vi "SA40144C.20210105.vi"() -> ()   [LabVIEW 2020]
uses:
  <vilib>/Analysis/baseanly.llb/Mean (DBL).vi
  <userlib>/LevyLab/LV to ITX/Data/Data.lvclass
  <userlib>/LevyLab/XY Utilities/xy_utilities.lvlib
  <vilib>/Analysis/NI_AALBase.lvlib
panel:
  in  "Array":path[](array[path])=[path "G:/My Drive/ansom/Data/PPMS 2/SA40144C.20210105/01 - Vacuum Thermal Decay/SA40144C.20210105.275K.dat", path "G:/My Drive/ansom/Data/PPMS 2/SA40144C.20210105/01 - Vacuum Thermal Decay/SA40144C.20210105.280K.dat", path "G:/My Drive/ansom/Data/PPMS 2/SA40144C.20210105/01 - Vacuum Thermal Decay/SA40144C.20210105.285K.dat", path "G:/My Drive/ansom/Data/PPMS 2/SA40144C.20210105/01 - Vacuum Thermal Decay/SA40144C.20210105.295K.dat", path "G:/My Drive/ansom/Data/PPMS 2/SA40144C.20210105/01 - Vacuum Thermal Decay/SA40144C.20210105.310K.dat", path "G:/My Drive/ansom/Data/PPMS 2/SA40144C.20210105/01 - Vacuum Thermal Decay/SA40144C.20210105.315K.dat", path "G:/My Drive/ansom/Data/PPMS 2/SA40144C.20210105/01 - Vacuum Thermal Decay/SA40144C.20210105.320K.dat", path "G:/My Drive/ansom/Data/PPMS 2/SA40144C.20210105/01 - Vacuum Thermal Decay/SA40144C.20210105.325K.dat", path "G:/My Drive/ansom/Data/PPMS 2/SA40144C.20210105/01 - Vacuum Thermal Decay/SA40144C.20210105.330K.dat", path "G:/My Drive/ansom/Data/PPMS 2/SA40144C.20210105/01 - Vacuum Thermal Decay/SA40144C.20210105.335K.dat", path "G:/My Drive/ansom/Data/PPMS 2/SA40144C.20210105/01 - Vacuum Thermal Decay/SA40144C.20210105.340K.dat", path "G:/My Drive/ansom/Data/PPMS 2/SA40144C.20210105/01 - Vacuum Thermal Decay/SA40144C.20210105.345K.dat", path "G:/My Drive/ansom/Data/PPMS 2/SA40144C.20210105/01 - Vacuum Thermal Decay/SA40144C.20210105.350K.dat"]
  in  "Temps to keep (Lifespan)":i32=26
  out "Lifespan vs Temp (hrs)":cluster{i32[], dbl[]}[](graph)
  out "E_a":dbl[](array[numeric])
  out "Arrhenius":T1(graph)
  in  "Temps to keep (Arrhenius fit)":i32=26
  out "G2T vs t":T1(graph)
  out "G4T vs t":T1(graph)
  out "G2T vs t 2D":T1(graph)
  out "G4T vs t  2D":T1(graph)
  in  "Source Voltage":dbl=0.01
  in  "Init Temp":i32=275
  in  "Temp Step":i32=5
  in  "Final Temp":i32=400
  in  "Trimming":i32=400
  in  "Update":bool
  in  "OK":bool
  out "error out":errorcluster
  in  "error in (no error)":errorcluster
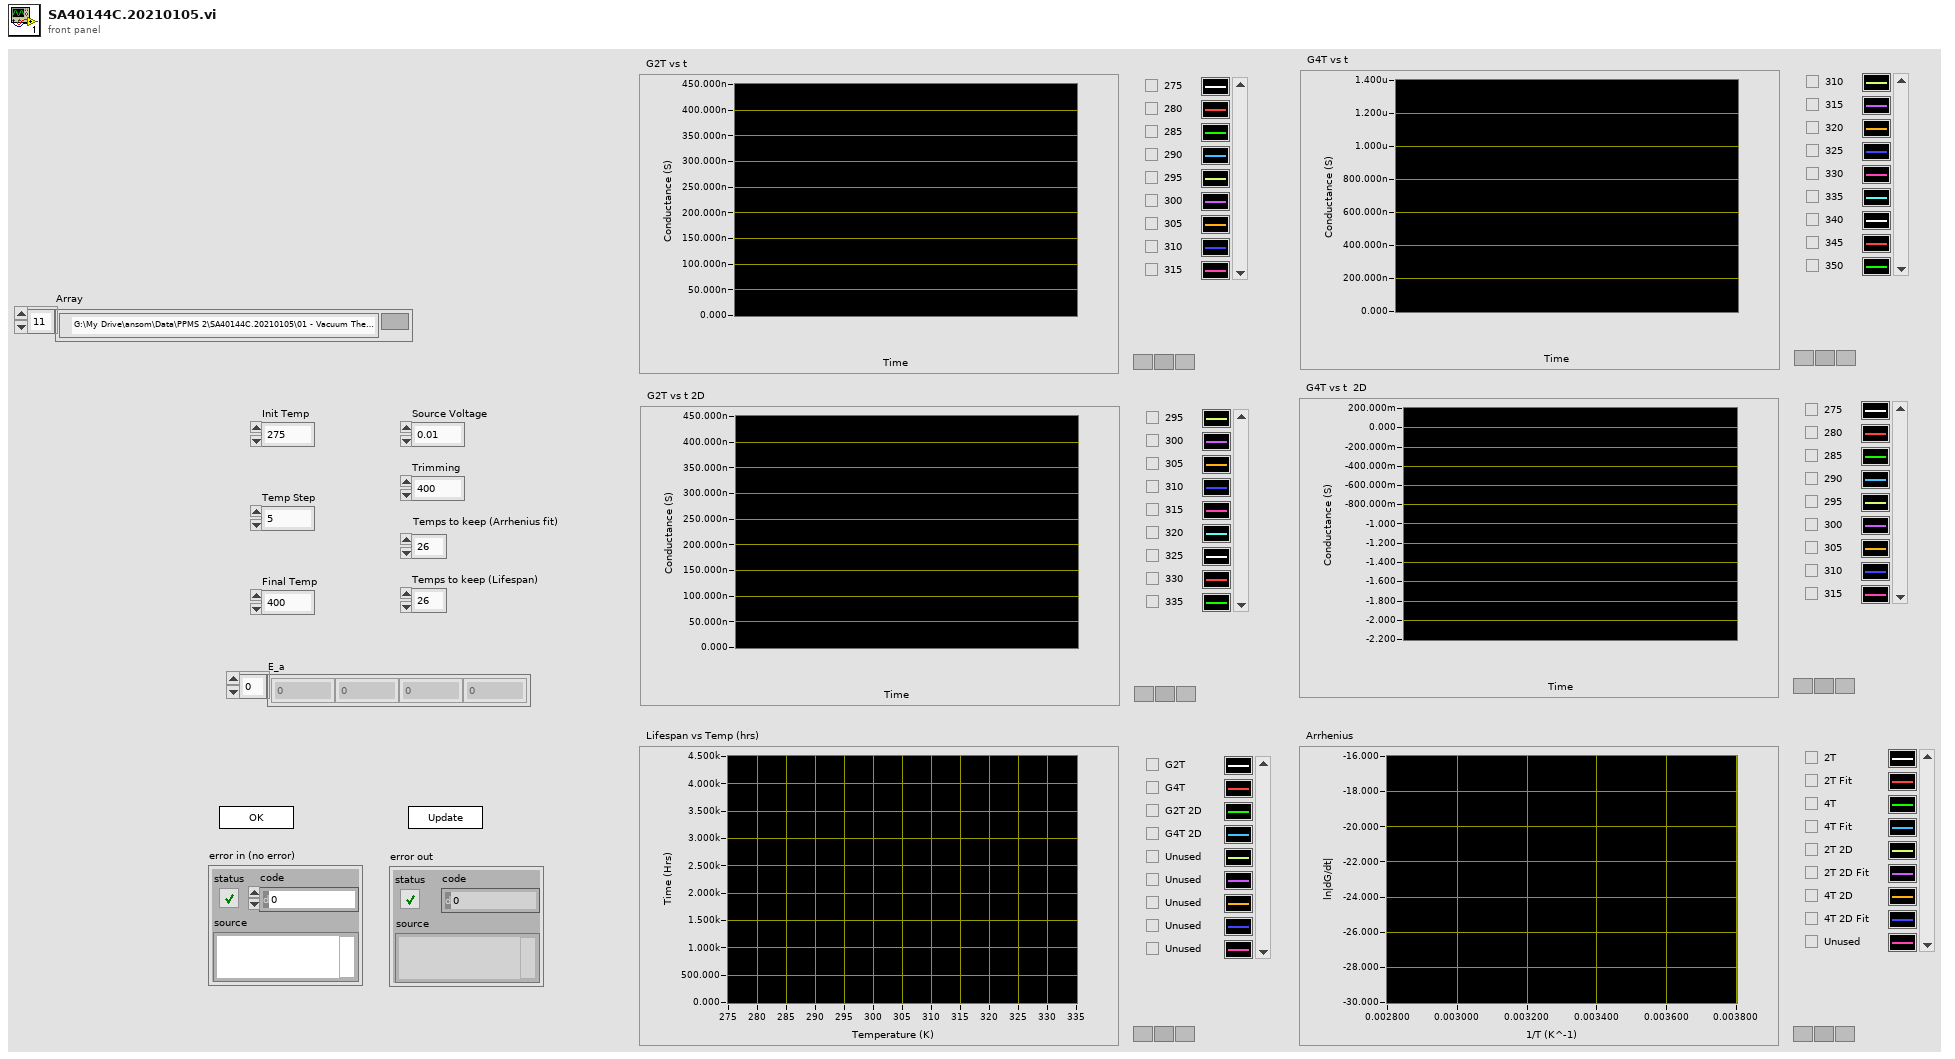
[diagram p1: front panel]
types:
  T1 = cluster{"Data":dbl[], "Best Exponential Fit":dbl[]}[]
  T2 = enum32{"Invalid", "Standard", "Closed", "Hidden", "Minimized", "Maximized"}
  T3 = enum32{"invalid app kind", "Development System", "Run Time System", "Student Edition", "Embedded LabVIEW", "Evaluation", "Custom"}
  T4 = cluster{"Core":cluster{"Current VI Reference":refnum<vi>, "Close Panel on Exit?":bool}, "G2T 1D":cluster{dbl[], dbl[]}[], "G4T 1D":cluster{dbl[], dbl[]}[], "G2T 2D":cluster{dbl[], dbl[]}[], "G4T 2D":cluster{dbl[], dbl[]}[], "Source Voltage":dbl, "Final Temp":i32, "Init Temp":i32, "Temp Step":i32, "Trimming":i32, "Array":path[], "Temp Array":dbl[]}
  T5 = cluster{"Current VI Reference":refnum<vi>, "Close Panel on Exit?":bool}
  T6 = typedef "Data.lvclass/Dictionary--cluster.ctl" = cluster{"key":string, "value":variant}
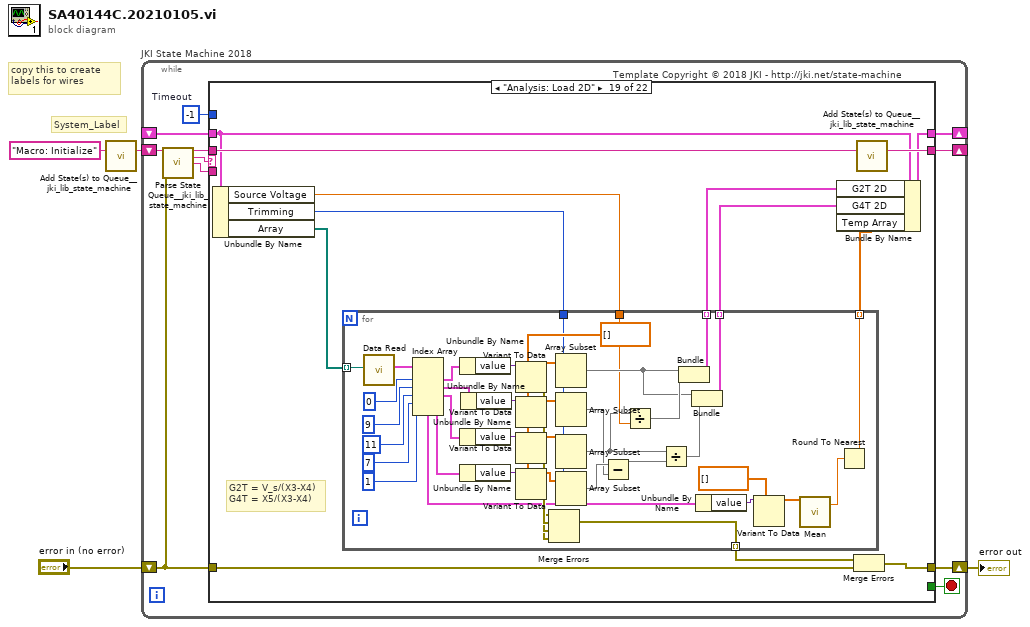
[diagram p0: block diagram]
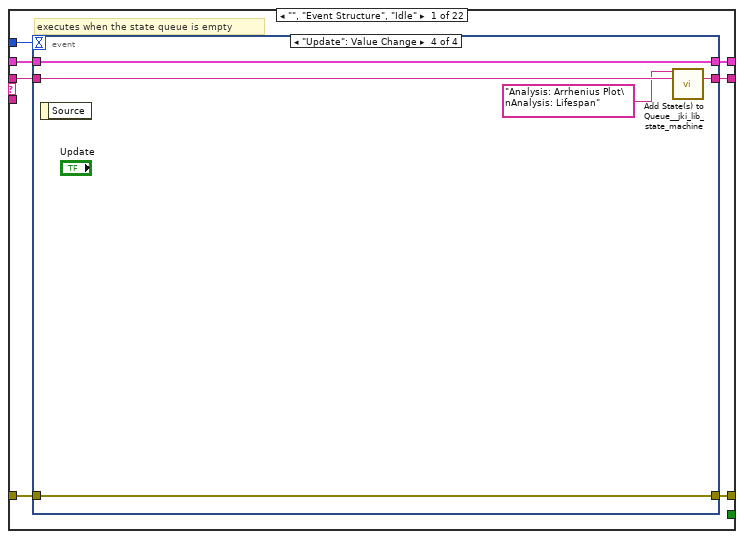
[diagram p2: hidden frame]
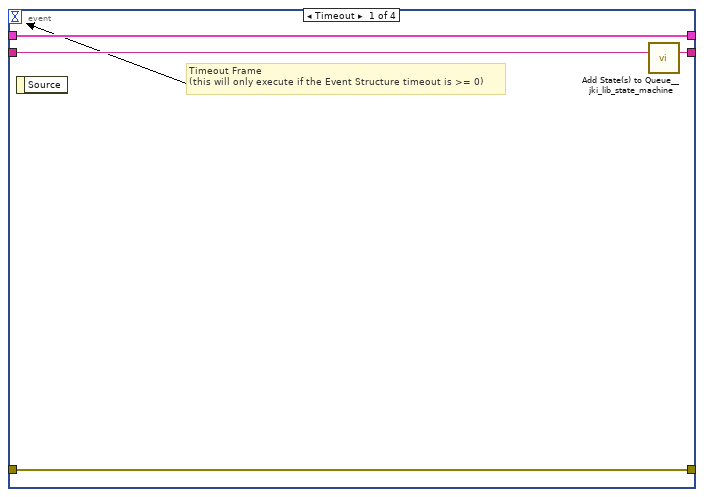
[diagram p3: hidden frame]
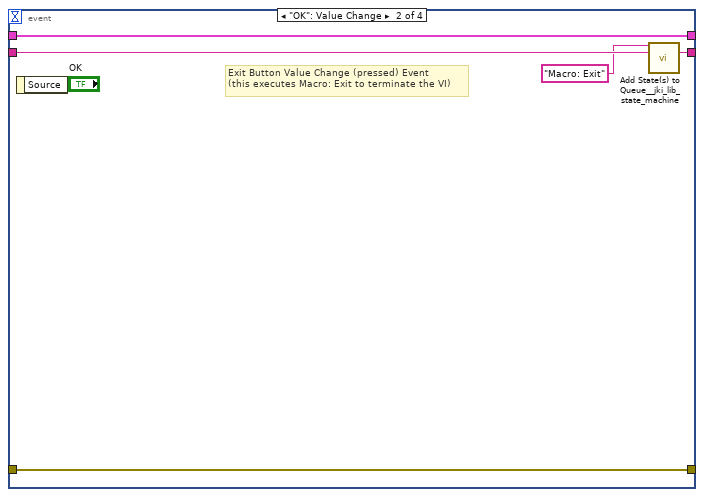
[diagram p4: hidden frame]
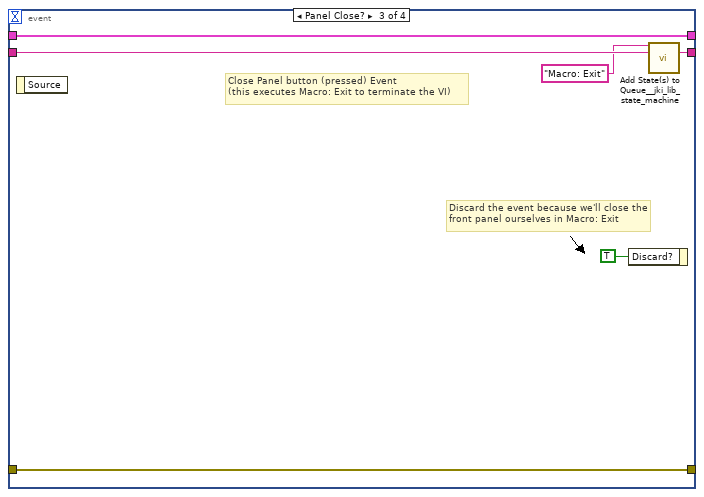
[diagram p5: hidden frame]
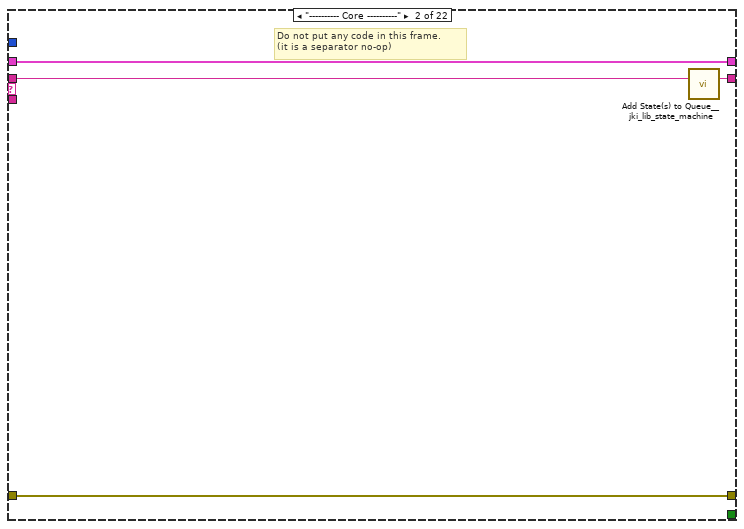
[diagram p6: hidden frame]
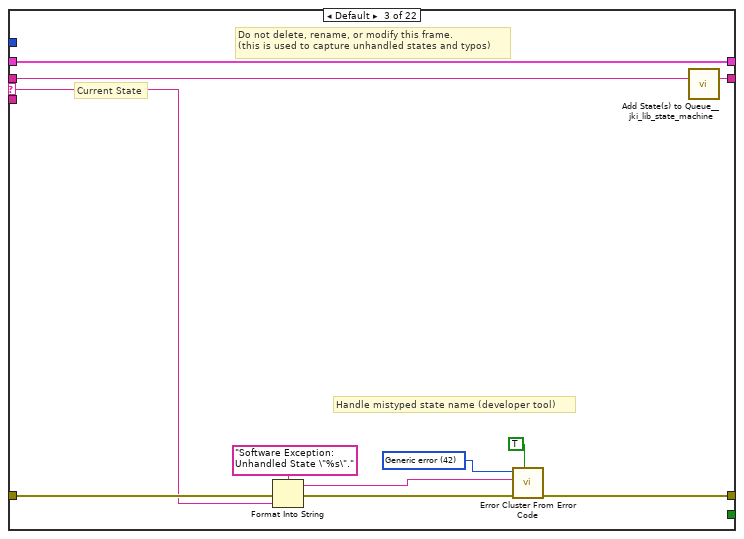
[diagram p7: hidden frame]
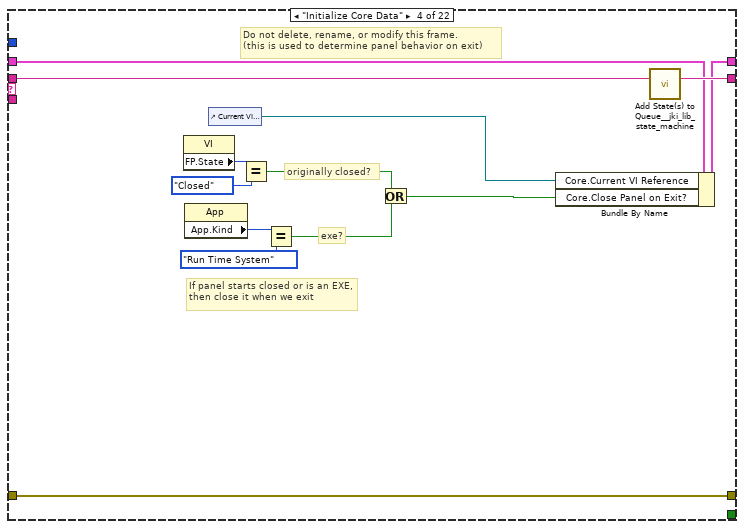
[diagram p8: hidden frame]
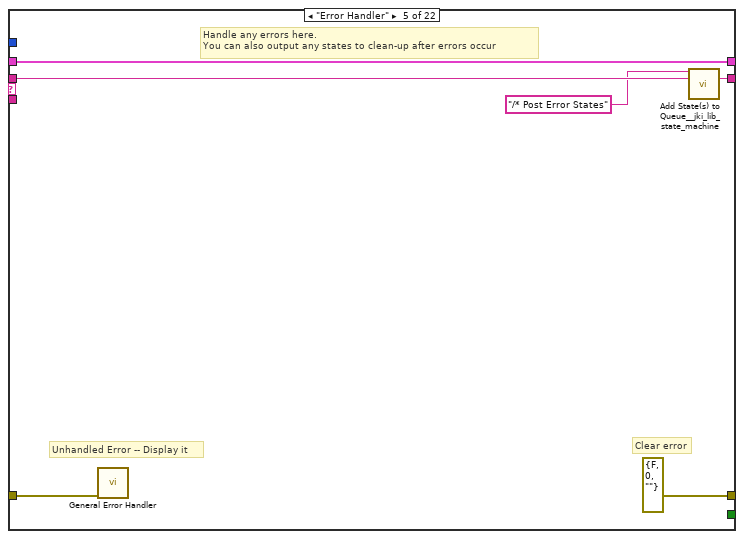
[diagram p9: hidden frame]
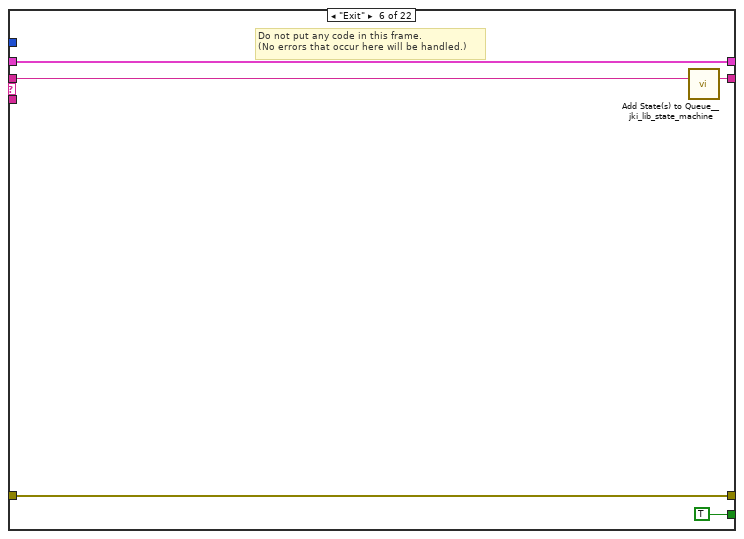
[diagram p10: hidden frame]
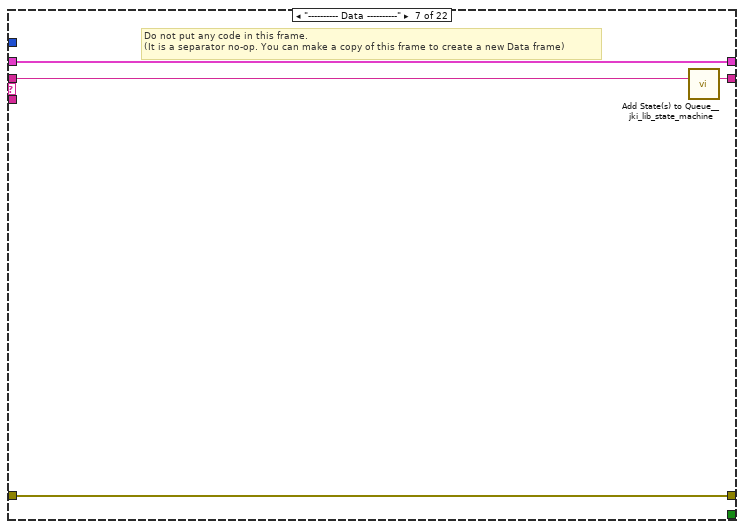
[diagram p11: hidden frame]
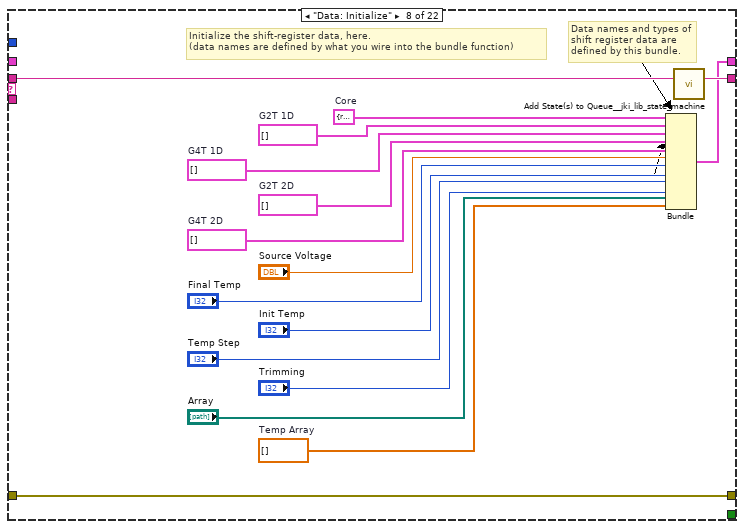
[diagram p12: hidden frame]
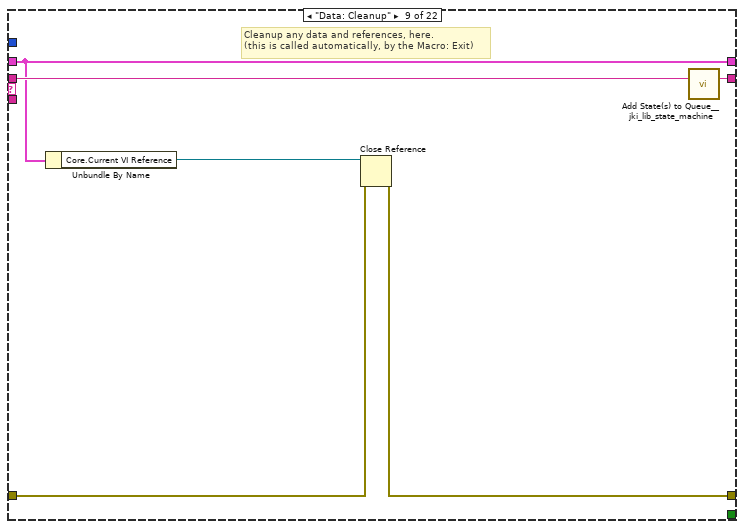
[diagram p13: hidden frame]
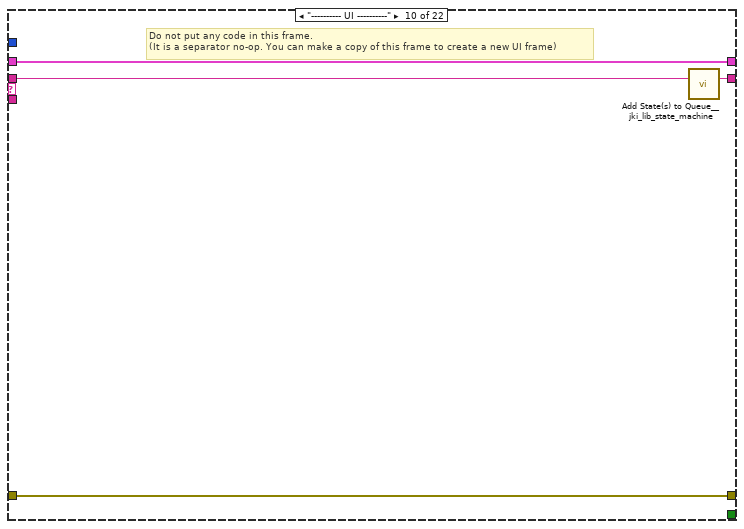
[diagram p14: hidden frame]
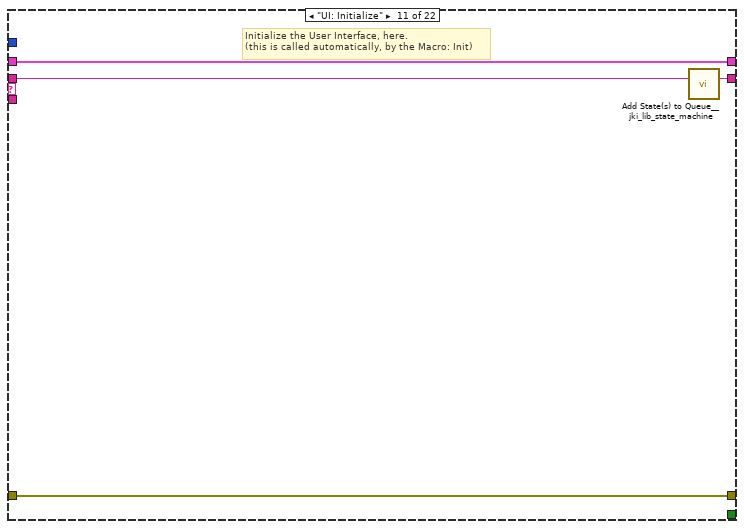
[diagram p15: hidden frame]
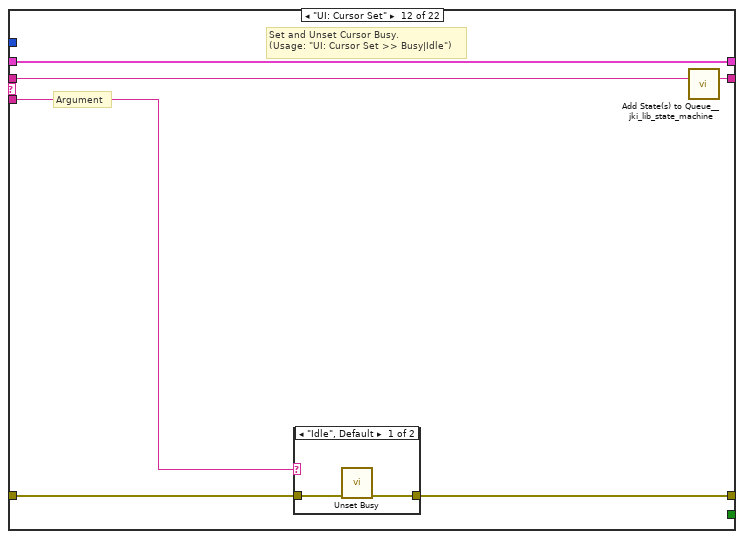
[diagram p16: hidden frame]
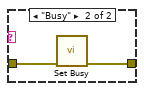
[diagram p17: hidden frame]
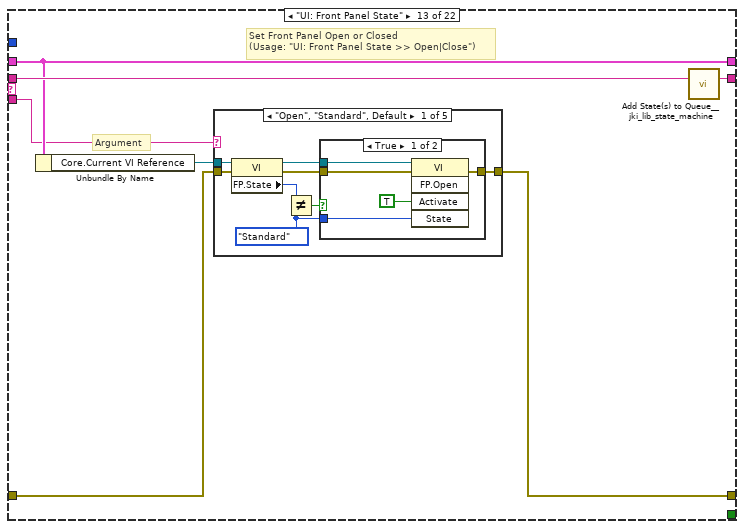
[diagram p18: hidden frame]
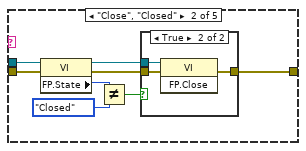
[diagram p20: hidden frame]
diagram:
  # "copy this to create labels for wires"
  # "System_Label"
  n1 = call <vilib>:"Add State(s) to Queue__jki_lib_state_machine.vi"("State(s) in (\"\")"="Macro: Initialize") -> ("States Out"=w4:string)  [unwired: 14 in]
  n2 = while "JKI State Machine 2018" {
    shift-right: [w8] -> _
    shift-left: _ -> [w7]
    shift-right: [w11] -> w1
    shift-left: "error in (no error)" -> [w5]
    shift-right: [w10] -> _
    shift-left: w4 -> [w12]
    stop <- w9 stop-if-true
    w6 = -1  # Timeout
    # "Template Copyright © 2018 JKI - http://jki.net/state-machine"
    n3 = call <vilib>:"Parse State Queue__jki_lib_state_machine.vi"("State Queue"=w12, "Error In (no error)"=w5) -> ("Remaining States"=w14:string, "Current State"=w15:string, "Arguments"=w13:string)  [unwired: 11 in]
    n4 = case shown="\"Analysis: Load 2D\"" w15 {
      selector: w15 -> [_ _ w47 _ _ _ _ _ _ _ _ _ _ _ _ _ _ _ _ _ _ _]
      tunnel: w14 -> [w22 w46 w51 w70 w76 w81 w85 w101 w107 w111 w115 w121 w132 w201 w206 w216 w220 w232 w280 w330 w369 w420]
      tunnel: w13 -> [_ _ _ _ _ _ _ _ _ _ _ w116 w126 _ _ _ _ _ _ _ _ _]
      tunnel: w7 -> [w20 w43 w49 w63 w73 w79 w82 _ w102 w108 w113 w119 w128 w198 w203 w213 w217 w226 w272 w327 w366 w400]
      tunnel: [w19 w44 w53 w67 errorcluster {"status"=FALSE, "code"=0, "source"=""} ("error out") w78 w83 w98 w103 w109 w112 w117 w129 w199 w204 w214 w218 w229 w278 w328 w367 w418] -> w11
      tunnel: w5 -> [w18 w44 w52 w67 w72 w78 w83 w98 w104 w109 w112 w118 w130 w199 w204 w214 w218 w230 w277 w328 w367 w418]
      tunnel: [w21 w45 w50 w69 w75 w80 w84 w100 w106 w110 w114 w120 w131 w200 w205 w215 w219 w231 w279 w329 w368 w419] -> w10
      tunnel: [_ _ _ _ _ TRUE _ _ _ _ _ _ _ _ _ _ _ _ _ _ _ _] -> w9
      tunnel: [w17 w43 w49 w68 w73 w79 w82 w99 w102 w108 w113 w119 w128 w198 w203 w213 w217 w227 w273 w327 w366 w400] -> w8
      tunnel: w6 -> [w16 _ _ _ _ _ _ _ _ _ _ _ _ _ _ _ _ _ _ _ _ _]
      frame "", "Event Structure", "Idle" {
        # "executes when the state queue is empty"
        n5 = event shown="[3] \"Update\": Value Change" {
          selector: _ -> [_ _ _ _]
          dyn-events: _ -> [_ _ _ _]
          timeout: w16 -> [_ _ _ _]
          tunnel: w22 -> [w26 w31 w37 w41]
          tunnel: [w25 w30 w36 w40] -> w21
          tunnel: w20 -> [w23 w28 w34 w42]
          tunnel: [w24 w29 w35 w38] -> w19
          tunnel: w18 -> [w24 w29 w35 w38]
          tunnel: [w23 w28 w34 w42] -> w17
          event Timeout {
            # "Timeout Frame\n(this will only execute if the Event Structure timeout is >= 0)"
            n6 = event-data() -> ()  [unwired: 1 in, 1 out]
            n7 = call <vilib>:"Add State(s) to Queue__jki_lib_state_machine.vi"("State(s) in (\"\")"=w26) -> ("States Out"=w25:string)  [unwired: 14 in]
          }
          event "OK": Value Change {
            # "Exit Button Value Change (pressed) Event\n(this executes Macro: Exit to terminate the VI)"
            n8 = event-data() -> ()  [unwired: 1 in, 1 out]
            n9 = call <vilib>:"Add State(s) to Queue__jki_lib_state_machine.vi"("State(s) in Front (\"\")"="Macro: Exit", "State(s) in (\"\")"=w31) -> ("States Out"=w30:string)  [unwired: 13 in]
          }
          event Panel Close? {
            # "Discard the event because we'll close the front panel ourselves in Macro: Exit"
            # "Close Panel button (pressed) Event\n(this executes Macro: Exit to terminate the VI)"
            n10 = event-data() -> ()  [unwired: 1 in, 1 out]
            n11 = event-data("Discard?"=TRUE) -> ()  [unwired: 1 in, 1 out]
            n12 = call <vilib>:"Add State(s) to Queue__jki_lib_state_machine.vi"("State(s) in Front (\"\")"="Macro: Exit", "State(s) in (\"\")"=w37) -> ("States Out"=w36:string)  [unwired: 13 in]
          }
          event "Update": Value Change {
            n13 = event-data() -> ()  [unwired: 1 in, 1 out]
            n14 = call <vilib>:"Add State(s) to Queue__jki_lib_state_machine.vi"("State(s) in Front (\"\")"="Analysis: Arrhenius Plot\nAnalysis: Lifespan" ("State(s) in Front (\"\")"), "State(s) in (\"\")"=w41) -> ("States Out"=w40:string)  [unwired: 13 in]
          }
        }
      }
      frame "---------- Core ----------" {
        # "Do not put any code in this frame.\n(it is a separator no-op)"
        n15 = call <vilib>:"Add State(s) to Queue__jki_lib_state_machine.vi"("State(s) in (\"\")"=w46) -> ("States Out"=w45:string)  [unwired: 14 in]
      }
      frame Default {
        w56 = 42 items=["No error", "Argument error", "Memory is full", "Out of zone", "End of file", "File already open", "Generic file I/O error", "File not found", "File permission error", "Disk is full", "Duplicate path", "Too many files open", "System feature not enabled", "Resource file not found", "Cannot add resource", "Resource not found", "Image not found", "Image memory error", "Pen does not exist", "Config type invalid", "Config token not found", "Config parse error", "Config memory error", "Bad external code format", "Bad external code offset", "External code not present", "Null window", "Destroy window error", "Null menu", "Print aborted", "Bad print record", "Print driver error", "Windows error during printing", "Memory error during printing", "Print dialog error", "Generic print error", "Invalid device refnum", "Device not found", "Device parameter error", "Device unit error", "Cannot open device", "Device call aborted", "Generic error", "Cancelled by user", "Object ID too low", "Object ID too high", "Object not in heap", "Unknown heap", "Unknown object (invalid DefProc)", "Unknown object (DefProc not in table)", "Message out of range", "Invalid (null) method", "Unknown message", "Manager call not supported", "Bad address", "Network operation in progress", "Network operation timed out", "Connection is busy", "Network attribute not supported", "Network error", "Address in use", "System out of memory", "Connection aborted", "Connection refused", "Not connected", "Already connected", "Connection closed", "Initialization error (interapplication manager)", "Bad occurrence", "Wait on unbound occurrence handler", "Occurrence queue overflow", "Datalog type conflict", "Unused", "Unrecognized type (interapplication manager)", "Memory corrupt", "Failed to make temporary DLL", "Old CIN version", "Drag socket not found", "Failed to load drop-object", "Failed to register OLE object", "Failed to release OLE object", "Format specifier type mismatch", "Unknown format specifier", "Too few format specifiers", "Too many format specifiers", "Scan failed", "Newer CIN version", "Error converting to variant", "Runtime menu error", "Password tampered", "Variant attribute not found", "Incompatible variant data type", "Event data is not available", "Event Store is not present", "Occurrence is not found", "Event Queue is not created", "Event info is not available", "Refnum passed is NULL", "Error retrieving Class GUID", "Error retrieving CoClass GUID", "Error retrieving TypeLib GUID.", "Bad built application magic bytes.", "Specific driver is different from the specific driver associated with the Logical Name.", "There is no session opened to the class driver.", "Max Error", "MAX - Error with config objects", "MAX - Error loading configuration", "MAX - Group not supported"]
        # "Current State"
        # "Do not delete, rename, or modify this frame.\n(this is used to capture unhandled states and typos)"
        # "Handle mistyped state name (developer tool)"
        n16 = Format Into String(format string="Software Exception: Unhandled State \"%s\"." ("message"), error in=w52, w47) -> (resulting string=w55:string, error out=w54:errorcluster)  [unwired: 1 in]
        n17 = call <vilib>:"Error Cluster From Error Code.vi"("show call chain? (False)"=TRUE, "error in (no error)"=w54, "error message (\"\")"=w55, "error code (0)"=w56) -> ("error out"=w53:errorcluster)  [unwired: 5 in]
        n18 = call <vilib>:"Add State(s) to Queue__jki_lib_state_machine.vi"("State(s) in (\"\")"=w51) -> ("States Out"=w50:string)  [unwired: 14 in]
      }
      frame "Initialize Core Data" {
        # "Do not delete, rename, or modify this frame.\n(this is used to determine panel behavior on exit)"
        # "originally closed?"
        # "exe?"
        # "If panel starts closed or is an EXE, then close it when we exit"
        n19 = property class="VI"() -> ("FP.State"=w60:T2)  [unwired: 2 in, 2 out]
        n20 = property class="App"() -> ("App.Kind"=w66:T3)  [unwired: 2 in, 2 out]
        n21 = control-ref of="Current VI Reference"() -> (w61:refnum<vi>)
        n22 = Equal?(x=w60, y=T2."Closed" ("Front Panel Window:State")) -> (x = y?=w58:bool)
        n23 = Equal?(x=w66, y=T3."Run Time System" ("Application:Kind")) -> (x = y?=w64:bool)
        n24 = Or(x=w58, y=w64) -> (x .or. y?=w62:bool)
        n25 = Bundle By Name(cluster=w63, "Core.Current VI Reference"=w61, "Core.Close Panel on Exit?"=w62) -> (w68:T4)
        n26 = call <vilib>:"Add State(s) to Queue__jki_lib_state_machine.vi"("State(s) in (\"\")"=w70) -> ("States Out"=w69:string)  [unwired: 14 in]
      }
      frame "Error Handler" {
        # "Unhandled Error -- Display it"
        # "Handle any errors here.\nYou can also output any states to clean-up after errors occur"
        # "Clear error"
        n27 = call <vilib>:"General Error Handler.vi"("error in (no error)"=w72) -> ()  [unwired: 10 in, 5 out]
        n28 = call <vilib>:"Add State(s) to Queue__jki_lib_state_machine.vi"("State(s) in Front (\"\")"="/* Post Error States", "State(s) in (\"\")"=w76) -> ("States Out"=w75:string)  [unwired: 13 in]
      }
      frame "Exit" {
        # "Do not put any code in this frame.\n(No errors that occur here will be handled.)"
        n29 = call <vilib>:"Add State(s) to Queue__jki_lib_state_machine.vi"("State(s) in (\"\")"=w81) -> ("States Out"=w80:string)  [unwired: 14 in]
      }
      frame "---------- Data ----------" {
        # "Do not put any code in this frame.\n(It is a separator no-op. You can make a copy of this frame to create a new Data frame)"
        n30 = call <vilib>:"Add State(s) to Queue__jki_lib_state_machine.vi"("State(s) in (\"\")"=w85) -> ("States Out"=w84:string)  [unwired: 14 in]
      }
      frame "Data: Initialize" {
        w86 = dbl[] []  # Temp Array
        w95 = cluster{dbl[], dbl[]}[] []  # G4T 2D
        w94 = cluster{dbl[], dbl[]}[] []  # G2T 2D
        w93 = cluster{dbl[], dbl[]}[] []  # G4T 1D
        w92 = cluster{dbl[], dbl[]}[] []  # G2T 1D
        w97 = T5 {"Current VI Reference"=refnum, "Close Panel on Exit?"=FALSE}  # Core
        # "Data names and types of shift register data are defined by this bundle."
        # "Initialize the shift-register data, here.\n(data names are defined by what you wire into the bundle function)"
        n31 = Bundle("Core"=w97, "G2T 1D"=w92, "G4T 1D"=w93, "G2T 2D"=w94, "G4T 2D"=w95, "Source Voltage"="Source Voltage", "Final Temp"="Final Temp", "Init Temp"="Init Temp", "Temp Step"="Temp Step", "Trimming"="Trimming", "Array"="Array", "Temp Array"=w86) -> (w99:T4)  [unwired: 1 in]
        n32 = call <vilib>:"Add State(s) to Queue__jki_lib_state_machine.vi"("State(s) in (\"\")"=w101) -> ("States Out"=w100:string)  [unwired: 14 in]
      }
      frame "Data: Cleanup" {
        # "Cleanup any data and references, here.\n(this is called automatically, by the Macro: Exit)"
        n33 = Unbundle By Name(w102) -> ("Core.Current VI Reference"=w105:refnum<vi>)
        n34 = Close Reference(reference=w105, error in (no error)=w104) -> (error out=w103:errorcluster)
        n35 = call <vilib>:"Add State(s) to Queue__jki_lib_state_machine.vi"("State(s) in (\"\")"=w107) -> ("States Out"=w106:string)  [unwired: 14 in]
      }
      frame "---------- UI ----------" {
        # "Do not put any code in this frame.\n(It is a separator no-op. You can make a copy of this frame to create a new UI frame)"
        n36 = call <vilib>:"Add State(s) to Queue__jki_lib_state_machine.vi"("State(s) in (\"\")"=w111) -> ("States Out"=w110:string)  [unwired: 14 in]
      }
      frame "UI: Initialize" {
        # "Initialize the User Interface, here.\n(this is called automatically, by the Macro: Init)"
        n37 = call <vilib>:"Add State(s) to Queue__jki_lib_state_machine.vi"("State(s) in (\"\")"=w115) -> ("States Out"=w114:string)  [unwired: 14 in]
      }
      frame "UI: Cursor Set" {
        # "Argument"
        # "Set and Unset Cursor Busy.\n(Usage: \"UI: Cursor Set >> Busy|Idle\")"
        n38 = case shown="\"Idle\", Default" w116 {
          tunnel: w118 -> [w123 w125]
          tunnel: [w122 w124] -> w117
          frame "Idle", Default {
            n39 = call <vilib>:"Unset Busy.vi"("error in (no error)"=w123) -> ("error out"=w122:errorcluster)  [unwired: 10 in]
          }
          frame "Busy" {
            n40 = call <vilib>:"Set Busy.vi"("error in (no error)"=w125) -> ("error out"=w124:errorcluster)  [unwired: 9 in, 1 out]
          }
        }
        n41 = call <vilib>:"Add State(s) to Queue__jki_lib_state_machine.vi"("State(s) in (\"\")"=w121) -> ("States Out"=w120:string)  [unwired: 14 in]
      }
      frame "UI: Front Panel State" {
        # "Argument"
        # "Set Front Panel Open or Closed\n(Usage: \"UI: Front Panel State >> Open|Close\")"
        n42 = Unbundle By Name(w128) -> ("Core.Current VI Reference"=w127:refnum<vi>)
        n43 = case shown="\"Open\", \"Standard\", Default" w126 {
          tunnel: w130 -> [w138 w153 w164 w177 w190]
          tunnel: [w140 w154 w166 w179 w192] -> w129
          tunnel: w127 -> [w139 w151 w165 w178 w191]
          frame "Open", "Standard", Default {
            w133 = T2."Standard" ("State")
            n44 = property class="VI"(reference=w139, error in=w138) -> (reference out=w136:refnum<vi>, error out=w137:errorcluster, "FP.State"=w135:T2)
            n45 = Not Equal?(x=w135, y=w133) -> (x != y?=w134:bool)
            n46 = case shown="True" w134 {
              tunnel: [w144 w146] -> w140
              tunnel: w137 -> [w143 w146]
              tunnel: w136 -> [w142 _]
              tunnel: w133 -> [w141 _]
              frame True {
                n47 = invoke class="VI" method="FP.Open"(reference=w142, error in=w143, "Activate"=TRUE, "State"=w141) -> (error out=w144:errorcluster)  [unwired: 1 in, 4 out]
              }
              frame False {
              }
            }
          }
          frame "Close", "Closed" {
            n48 = property class="VI"(reference=w151, error in=w153) -> (reference out=w150:refnum<vi>, error out=w152:errorcluster, "FP.State"=w148:T2)
            n49 = Not Equal?(x=w148, y=T2."Closed" ("Front Panel Window:State")) -> (x != y?=w147:bool)
            n50 = case shown="True" w147 {
              tunnel: [w155 w158] -> w154
              tunnel: w152 -> [w155 w157]
              tunnel: w150 -> [_ w156]
              frame False {
              }
              frame True {
                n51 = invoke class="VI" method="FP.Close"(reference=w156, error in=w157) -> (error out=w158:errorcluster)  [unwired: 1 in, 2 out]
              }
            }
          }
          frame "Hidden", "Hide" {
            w159 = T2."Hidden" ("State")
            n52 = property class="VI"(reference=w165, error in=w164) -> (reference out=w162:refnum<vi>, error out=w163:errorcluster, "FP.State"=w161:T2)
            n53 = Not Equal?(x=w161, y=w159) -> (x != y?=w160:bool)
            n54 = case shown="True" w160 {
              tunnel: [w170 w171] -> w166
              tunnel: w163 -> [w169 w171]
              tunnel: w162 -> [w168 _]
              tunnel: w159 -> [w167 _]
              frame True {
                n55 = invoke class="VI" method="FP.Open"(reference=w168, error in=w169, "State"=w167) -> (error out=w170:errorcluster)  [unwired: 2 in, 4 out]
              }
              frame False {
              }
            }
          }
          frame "Minimize", "Minimized" {
            w172 = T2."Minimized" ("State")
            n56 = property class="VI"(reference=w178, error in=w177) -> (reference out=w175:refnum<vi>, error out=w176:errorcluster, "FP.State"=w174:T2)
            n57 = Not Equal?(x=w174, y=w172) -> (x != y?=w173:bool)
            n58 = case shown="True" w173 {
              tunnel: [w183 w184] -> w179
              tunnel: w176 -> [w182 w184]
              tunnel: w175 -> [w181 _]
              tunnel: w172 -> [w180 _]
              frame True {
                n59 = invoke class="VI" method="FP.Open"(reference=w181, error in=w182, "State"=w180) -> (error out=w183:errorcluster)  [unwired: 2 in, 4 out]
              }
              frame False {
              }
            }
          }
          frame "Maximize", "Maximized" {
            w185 = T2."Maximized" ("State")
            n60 = property class="VI"(reference=w191, error in=w190) -> (reference out=w188:refnum<vi>, error out=w189:errorcluster, "FP.State"=w187:T2)
            n61 = Not Equal?(x=w187, y=w185) -> (x != y?=w186:bool)
            n62 = case shown="True" w186 {
              tunnel: [w196 w197] -> w192
              tunnel: w189 -> [w195 w197]
              tunnel: w188 -> [w194 _]
              tunnel: w185 -> [w193 _]
              frame True {
                n63 = invoke class="VI" method="FP.Open"(reference=w194, error in=w195, "State"=w193) -> (error out=w196:errorcluster)  [unwired: 2 in, 4 out]
              }
              frame False {
              }
            }
          }
        }
        n64 = call <vilib>:"Add State(s) to Queue__jki_lib_state_machine.vi"("State(s) in (\"\")"=w132) -> ("States Out"=w131:string)  [unwired: 14 in]
      }
      frame "---------- Macro ----------" {
        # "Do not put any code in this frame.\n(It is a separator no-op. You can make a copy of this frame to create a new Macro frame)"
        n65 = call <vilib>:"Add State(s) to Queue__jki_lib_state_machine.vi"("State(s) in (\"\")"=w201) -> ("States Out"=w200:string)  [unwired: 14 in]
      }
      frame "Macro: Initialize" {
        # "Initialization Macro\n(This is called once, when the VI starts)"
        n66 = call <vilib>:"Add State(s) to Queue__jki_lib_state_machine.vi"("State(s) in Front (\"\")"="Data: Initialize\nInitialize Core Data\nUI: Initialize\nUI: Front Panel State >> Open\nAnalysis: Load 1D\nAnalysis: Load 2D\nAnalysis: Plot G vs t\nAnalysis: Arrhenius Plot\nAnalysis: Lifespan", "State(s) in (\"\")"=w206) -> ("States Out"=w205:string)  [unwired: 13 in]
      }
      frame "Macro: Exit" {
        # "Exit Macro\n(This is called once, when the VI exits)"
        n67 = Unbundle By Name(w213) -> ("Core.Close Panel on Exit?"=w212:bool)
        n68 = Select(t="UI: Front Panel State >> Close", s=w212, f="") -> (s? t:f=w209:string)
        n69 = call <vilib>:"Add State(s) to Queue__jki_lib_state_machine.vi"("State(s) in (\"\")"=w209, "State(s) at Back (\"\")"="Data: Cleanup\nExit") -> ("States Out"=w207:string)  [unwired: 13 in]
        n70 = call <vilib>:"Add State(s) to Queue__jki_lib_state_machine.vi"("State(s) in Front (\"\")"=w207, "State(s) in (\"\")"=w216) -> ("States Out"=w215:string)  [unwired: 13 in]
      }
      frame "---------- Analysis ----------" {
        # "Template Separator\n(You can make a copy of, or modify, this frame)"
        n71 = call <vilib>:"Add State(s) to Queue__jki_lib_state_machine.vi"("State(s) in (\"\")"=w220) -> ("States Out"=w219:string)  [unwired: 14 in]
      }
      frame "Analysis: Load 1D" {
        # "G2T = V_s/(X1-X7)\nG4T = X5/(X1-X7)"
        n72 = Unbundle By Name(w226) -> ("Source Voltage"=w225:dbl, "Trimming"=w222:i32, "Array"=w221:path[])
        n73 = for {
          tunnel: [w249] -> w228 mode=indexing
          tunnel: w225 -> [w234]
          tunnel: [w245] -> w224 mode=indexing
          tunnel: [w244] -> w223 mode=indexing
          tunnel: w221 -> [w235] mode=indexing
          tunnel: [w236] -> _
          tunnel: w222 -> [w236]
          w259 = dbl[] []
          n74 = call <userlib>:"Data Read.vi"("path"=w235) -> ("Data (Dictionary)"=w262:T6[])  [unwired: 7 in, 3 out]
          n75 = Index Array(array=w262, index #1=0, index #2=3, index #3=11 ("index"), index #4=15) -> (element #1=w254:T6, element #2=w253:T6, element #3=w252:T6, element #4=w251:T6)
          n76 = Unbundle By Name(w254) -> ("value"=w258:variant)
          n77 = Unbundle By Name(w252) -> ("value"=w256:variant)
          n78 = Unbundle By Name(w251) -> ("value"=w255:variant)
          n79 = Unbundle By Name(w253) -> ("value"=w257:variant)
          n80 = Variant To Data(type=w259, Variant=w258) -> (data=w240:dbl[], error out=w250:errorcluster)  [unwired: 1 in]
          n81 = Variant To Data(type=w259, Variant=w257) -> (data=w238:dbl[], error out=w265:errorcluster)  [unwired: 1 in]
          n82 = Variant To Data(type=w259, Variant=w256) -> (data=w241:dbl[], error out=w264:errorcluster)  [unwired: 1 in]
          n83 = Variant To Data(type=w259, Variant=w255) -> (data=w243:dbl[], error out=w263:errorcluster)  [unwired: 1 in]
          n84 = Merge Errors(w250, w265, w264, w263) -> (w249:errorcluster)
          n85 = Array Subset(array=w240, index=w236) -> (w239:dbl[])  [unwired: 1 in]
          n86 = Array Subset(array=w238, index=w236) -> (w237:dbl[])  [unwired: 1 in]
          n87 = Array Subset(array=w241, index=w236) -> (w233:dbl[])  [unwired: 1 in]
          n88 = Array Subset(array=w243, index=w236) -> (w242:dbl[])  [unwired: 1 in]
          n89 = Subtract(x=w242, y=w237) -> (x-y=w248:dbl[])
          n90 = Divide(x=w233, y=w234) -> (x/y=w246:dbl[])
          n91 = Divide(x=w233, y=w248) -> (x/y=w247:dbl[])
          n92 = Bundle(w239, w246) -> (w245:cluster{dbl[], dbl[]})  [unwired: 1 in]
          n93 = Bundle(w239, w247) -> (w244:cluster{dbl[], dbl[]})  [unwired: 1 in]
        }
        n94 = Merge Errors(w228, w230) -> (w229:errorcluster)
        n95 = call <vilib>:"Add State(s) to Queue__jki_lib_state_machine.vi"("State(s) in (\"\")"=w232) -> ("States Out"=w231:string)  [unwired: 14 in]
        n96 = Bundle By Name(cluster=w226, "G2T 1D"=w224, "G4T 1D"=w223) -> (w227:T4)
      }
      frame "Analysis: Load 2D" {
        # "G2T = V_s/(X3-X4)\nG4T = X5/(X3-X4)"
        n97 = Unbundle By Name(w272) -> ("Source Voltage"=w276:dbl, "Trimming"=w269:i32, "Array"=w270:path[])
        n98 = for {
          tunnel: [w304] -> w271 mode=indexing
          tunnel: w276 -> [w282]
          tunnel: [w300] -> w275 mode=indexing
          tunnel: [w299] -> w274 mode=indexing
          tunnel: w269 -> [w298]
          tunnel: w270 -> [w290] mode=indexing
          tunnel: [w283] -> w268 mode=indexing
          w314 = dbl[] []
          n99 = call <userlib>:"Data Read.vi"("path"=w290) -> ("Data (Dictionary)"=w317:T6[])  [unwired: 7 in, 3 out]
          n100 = Index Array(array=w317, index #1=0, index #2=9, index #3=11 ("index"), index #4=7, index #5=1 ("index")) -> (element #1=w309:T6, element #2=w308:T6, element #3=w307:T6, element #4=w306:T6, element #5=w288:T6)
          n101 = Unbundle By Name(w309) -> ("value"=w313:variant)
          n102 = Unbundle By Name(w307) -> ("value"=w311:variant)
          n103 = Unbundle By Name(w306) -> ("value"=w310:variant)
          n104 = Unbundle By Name(w308) -> ("value"=w312:variant)
          n105 = Variant To Data(type=w314, Variant=w313) -> (data=w294:dbl[], error out=w305:errorcluster)  [unwired: 1 in]
          n106 = Variant To Data(type=w314, Variant=w312) -> (data=w292:dbl[], error out=w320:errorcluster)  [unwired: 1 in]
          n107 = Variant To Data(type=w314, Variant=w311) -> (data=w295:dbl[], error out=w319:errorcluster)  [unwired: 1 in]
          n108 = Variant To Data(type=w314, Variant=w310) -> (data=w297:dbl[], error out=w318:errorcluster)  [unwired: 1 in]
          n109 = Merge Errors(w305, w320, w319, w318) -> (w304:errorcluster)
          n110 = Array Subset(array=w294, index=w298) -> (w293:dbl[])  [unwired: 1 in]
          n111 = Array Subset(array=w292, index=w298) -> (w291:dbl[])  [unwired: 1 in]
          n112 = Array Subset(array=w295, index=w298) -> (w281:dbl[])  [unwired: 1 in]
          n113 = Array Subset(array=w297, index=w298) -> (w296:dbl[])  [unwired: 1 in]
          n114 = Subtract(x=w296, y=w291) -> (x-y=w303:dbl[])
          n115 = Divide(x=w281, y=w282) -> (x/y=w301:dbl[])
          n116 = Divide(x=w281, y=w303) -> (x/y=w302:dbl[])
          n117 = Bundle(w293, w301) -> (w300:cluster{dbl[], dbl[]})  [unwired: 1 in]
          n118 = Bundle(w293, w302) -> (w299:cluster{dbl[], dbl[]})  [unwired: 1 in]
          n119 = Unbundle By Name(w288) -> ("value"=w287:variant)
          n120 = Variant To Data(type=dbl[] [], Variant=w287) -> (data=w285:dbl[])  [unwired: 1 in, 1 out]
          n121 = call-poly <vilib>:"Mean.vi"("X"=w285) -> ("mean"=w284:dbl)  [unwired: 1 out]
          n122 = Round To Nearest(number=w284) -> (nearest integer value=w283:dbl)
        }
        n123 = Bundle By Name(cluster=w272, "G2T 2D"=w275, "G4T 2D"=w274, "Temp Array"=w268) -> (w273:T4)
        n124 = Merge Errors(w271, w277) -> (w278:errorcluster)
        n125 = call <vilib>:"Add State(s) to Queue__jki_lib_state_machine.vi"("State(s) in (\"\")"=w280) -> ("States Out"=w279:string)  [unwired: 14 in]
      }
      frame "Analysis: Plot G vs t" {
        n126 = Unbundle By Name(w327) -> ("G2T 1D"=→"G2T vs t":cluster{dbl[], dbl[]}[], "G4T 1D"=→"G4T vs t":cluster{dbl[], dbl[]}[], "G2T 2D"=→"G2T vs t 2D":cluster{dbl[], dbl[]}[], "G4T 2D"=→"G4T vs t  2D":cluster{dbl[], dbl[]}[])
        n127 = call <vilib>:"Add State(s) to Queue__jki_lib_state_machine.vi"("State(s) in (\"\")"=w330) -> ("States Out"=w329:string)  [unwired: 14 in]
      }
      frame "Analysis: Arrhenius Plot" {
        n128 = Unbundle By Name(w366) -> ("G2T 1D"=w336:cluster{dbl[], dbl[]}[], "G4T 1D"=w335:cluster{dbl[], dbl[]}[], "G2T 2D"=w342:cluster{dbl[], dbl[]}[], "G4T 2D"=w344:cluster{dbl[], dbl[]}[], "Temp Array"=w332:dbl[])  [unwired: 1 out]
        n129 = call-poly <userlib>:"Linear Fit.vi"("XY-data"=w336) -> ("slopes"=w333:dbl[])  [unwired: 4 in, 6 out]
        n130 = call-poly <userlib>:"Linear Fit.vi"("XY-data"=w335) -> ("slopes"=w334:dbl[])  [unwired: 4 in, 6 out]
        n131 = call-poly <userlib>:"Linear Fit.vi"("XY-data"=w342) -> ("slopes"=w341:dbl[])  [unwired: 4 in, 6 out]
        n132 = call-poly <userlib>:"Linear Fit.vi"("XY-data"=w344) -> ("slopes"=w343:dbl[])  [unwired: 4 in, 6 out]
        n133 = Reciprocal(x=w332) -> (1/x=w331:dbl[])
        n134 = Absolute Value(x=w333) -> (abs(x)=w362:dbl[])
        n135 = Absolute Value(x=w334) -> (abs(x)=w363:dbl[])
        n136 = Absolute Value(x=w341) -> (abs(x)=w364:dbl[])
        n137 = Absolute Value(x=w343) -> (abs(x)=w365:dbl[])
        n138 = Natural Logarithm(1:w362) -> (0:w356:dbl[])
        n139 = Natural Logarithm(1:w363) -> (0:w355:dbl[])
        n140 = Natural Logarithm(1:w364) -> (0:w354:dbl[])
        n141 = Natural Logarithm(1:w365) -> (0:w353:dbl[])
        n142 = Array Subset(array=w356, length="Temps to keep (Arrhenius fit)") -> (w351:dbl[])  [unwired: 1 in]
        n143 = Array Subset(array=w355, length="Temps to keep (Arrhenius fit)") -> (w350:dbl[])  [unwired: 1 in]
        n144 = Array Subset(array=w354, length="Temps to keep (Arrhenius fit)") -> (w349:dbl[])  [unwired: 1 in]
        n145 = Array Subset(array=w353, length="Temps to keep (Arrhenius fit)") -> (w348:dbl[])  [unwired: 1 in]
        n146 = Array Subset(array=w331, length="Temps to keep (Arrhenius fit)") -> (w347:dbl[])  [unwired: 1 in]
        n147 = Bundle(w347, w351) -> (w359:cluster{dbl[], dbl[]})  [unwired: 1 in]
        n148 = Bundle(w347, w350) -> (w361:cluster{dbl[], dbl[]})  [unwired: 1 in]
        n149 = Bundle(w347, w349) -> (w360:cluster{dbl[], dbl[]})  [unwired: 1 in]
        n150 = Bundle(w347, w348) -> (w358:cluster{dbl[], dbl[]})  [unwired: 1 in]
        n151 = Build Array(w359, w361, w360, w358) -> (w340:cluster{dbl[], dbl[]}[])
        n152 = call-poly <userlib>:"Linear Fit.vi"("XY-data"=w340) -> ("Best Fits"=w339:cluster{"X-array":dbl[], "Y-array":dbl[]}[], "XY-data out"=w338:cluster{"X-array":dbl[], "Y-array":dbl[]}[], "slopes"=w337:dbl[])  [unwired: 4 in, 4 out]
        n153 = Multiply(x=w337, y=8.617333e-05) -> (x*y=→"E_a":dbl[])
        n154 = Interleave 1D Arrays(w338, w339) -> (→"Arrhenius":cluster{"X-array":dbl[], "Y-array":dbl[]}[])
        n155 = call <vilib>:"Add State(s) to Queue__jki_lib_state_machine.vi"("State(s) in (\"\")"=w369) -> ("States Out"=w368:string)  [unwired: 14 in]
      }
      frame "Analysis: Lifespan" {
        w378 = 3600
        # "Template Separator\n(You can make a copy of, or modify, this frame)"
        n156 = Unbundle By Name(w400) -> ("G2T 1D"=w417:cluster{dbl[], dbl[]}[], "G4T 1D"=w416:cluster{dbl[], dbl[]}[], "G2T 2D"=w415:cluster{dbl[], dbl[]}[], "G4T 2D"=w414:cluster{dbl[], dbl[]}[], "Final Temp"=w411:i32, "Init Temp"=w399:i32, "Temp Step"=w398:i32)  [unwired: 1 out]
        n157 = Subtract(x=w411, y=w399) -> (x-y=w412:i32)
        n158 = Divide(x=w412, y=w398) -> (x/y=w413:dbl)
        n159 = Increment(x=w413) -> (x+1=w397:dbl)
        n160 = for {
          N: w397 -> [_]
          tunnel: w399 -> [w435]
          tunnel: w398 -> [w434]
          tunnel: [w433] -> w396 mode=indexing
          i -> [w436]
          n161 = Multiply(x=w434, y=w436) -> (x*y=w437:i32)
          n162 = Add(x=w435, y=w437) -> (x+y=w433:i32)
        }
        n163 = call <userlib>:"Linear Fit (multiple).vi"("XY-data"=w417) -> ("XY-data out"=w391:cluster{"X-array":dbl[], "Y-array":dbl[]}[], "slopes"=w394:dbl[])  [unwired: 4 in, 5 out]
        n164 = call <userlib>:"Linear Fit (multiple).vi"("XY-data"=w416) -> ("XY-data out"=w390:cluster{"X-array":dbl[], "Y-array":dbl[]}[], "slopes"=w393:dbl[])  [unwired: 4 in, 5 out]
        n165 = call <userlib>:"Linear Fit (multiple).vi"("XY-data"=w415) -> ("XY-data out"=w389:cluster{"X-array":dbl[], "Y-array":dbl[]}[], "slopes"=w392:dbl[])  [unwired: 4 in, 5 out]
        n166 = call <userlib>:"Linear Fit (multiple).vi"("XY-data"=w414) -> ("XY-data out"=w388:cluster{"X-array":dbl[], "Y-array":dbl[]}[], "slopes"=w395:dbl[])  [unwired: 4 in, 5 out]
        n167 = for {
          tunnel: w391 -> [w429] mode=indexing
          tunnel: w390 -> [w430] mode=indexing
          tunnel: w389 -> [w431] mode=indexing
          tunnel: w388 -> [w432] mode=indexing
          tunnel: [w424] -> w387 mode=indexing
          tunnel: [w423] -> w386 mode=indexing
          tunnel: [w422] -> w385 mode=indexing
          tunnel: [w421] -> w384 mode=indexing
          n168 = Unbundle(w429) -> ("Y-array"=w425:dbl[])  [unwired: 1 out]
          n169 = Unbundle(w430) -> ("Y-array"=w426:dbl[])  [unwired: 1 out]
          n170 = Unbundle(w431) -> ("Y-array"=w427:dbl[])  [unwired: 1 out]
          n171 = Unbundle(w432) -> ("Y-array"=w428:dbl[])  [unwired: 1 out]
          n172 = call-poly <vilib>:"Mean.vi"("X"=w428) -> ("mean"=w421:dbl)  [unwired: 1 out]
          n173 = call-poly <vilib>:"Mean.vi"("X"=w427) -> ("mean"=w422:dbl)  [unwired: 1 out]
          n174 = call-poly <vilib>:"Mean.vi"("X"=w426) -> ("mean"=w423:dbl)  [unwired: 1 out]
          n175 = call-poly <vilib>:"Mean.vi"("X"=w425) -> ("mean"=w424:dbl)  [unwired: 1 out]
        }
        n176 = Divide(x=w387, y=w394) -> (x/y=w382:dbl[])
        n177 = Divide(x=w386, y=w393) -> (x/y=w381:dbl[])
        n178 = Divide(x=w385, y=w392) -> (x/y=w380:dbl[])
        n179 = Divide(x=w384, y=w395) -> (x/y=w379:dbl[])
        n180 = Divide(x=w382, y=w378) -> (x/y=w374:dbl[])
        n181 = Divide(x=w381, y=w378) -> (x/y=w375:dbl[])
        n182 = Divide(x=w380, y=w378) -> (x/y=w376:dbl[])
        n183 = Divide(x=w379, y=w378) -> (x/y=w377:dbl[])
        n184 = Array Subset(array=w374, length="Temps to keep (Lifespan)") -> (w405:dbl[])  [unwired: 1 in]
        n185 = Array Subset(array=w375, length="Temps to keep (Lifespan)") -> (w404:dbl[])  [unwired: 1 in]
        n186 = Array Subset(array=w376, length="Temps to keep (Lifespan)") -> (w403:dbl[])  [unwired: 1 in]
        n187 = Array Subset(array=w377, length="Temps to keep (Lifespan)") -> (w402:dbl[])  [unwired: 1 in]
        n188 = Array Subset(array=w396, length="Temps to keep (Lifespan)") -> (w401:i32[])  [unwired: 1 in]
        n189 = Absolute Value(x=w405) -> (abs(x)=w370:dbl[])
        n190 = Absolute Value(x=w404) -> (abs(x)=w371:dbl[])
        n191 = Absolute Value(x=w403) -> (abs(x)=w372:dbl[])
        n192 = Absolute Value(x=w402) -> (abs(x)=w373:dbl[])
        n193 = Bundle(w401, w370) -> (w408:cluster{i32[], dbl[]})  [unwired: 1 in]
        n194 = Bundle(w401, w371) -> (w410:cluster{i32[], dbl[]})  [unwired: 1 in]
        n195 = Bundle(w401, w372) -> (w409:cluster{i32[], dbl[]})  [unwired: 1 in]
        n196 = Bundle(w401, w373) -> (w407:cluster{i32[], dbl[]})  [unwired: 1 in]
        n197 = Build Array(w408, w410, w409, w407) -> (→"Lifespan vs Temp (hrs)":cluster{i32[], dbl[]}[])
        n198 = call <vilib>:"Add State(s) to Queue__jki_lib_state_machine.vi"("State(s) in (\"\")"=w420) -> ("States Out"=w419:string)  [unwired: 14 in]
      }
    }
  }
  "error out" <- w1
